vi "Angle Rotation (array).vi"(7 "angle units":T1 items=["radian in, radian out", "radian in, degree out", "degree in, degree out", "degree in, radian out"], 9 "rotated angle range":T2=1 items=["none", "-180 to 180 (-pi to pi)", "0 to 360 (0 to 2pi)"], 10 "Counterclockwise Rotation":dbl[](array[numeric]), 11 "Angle":dbl[](array[numeric])) -> (0 "error":i32, 3 "Rotated Angle":dbl[](array[numeric]))   [LabVIEW 2017, in "NI_AAL_Angle.lvlib"]
doc: "Rotates the input angle counterclockwise.\n\nWire data to the angle input to determine the polymorphic instance to use or manually select the instance."
uses:
  <vilib>/Analysis/NI_AAL_Angle.lvlib
  <vilib>/Analysis/coordinate.llb/Angle Range (Degree).ctl
  <vilib>/Analysis/coordinate.llb/Angle Units.ctl
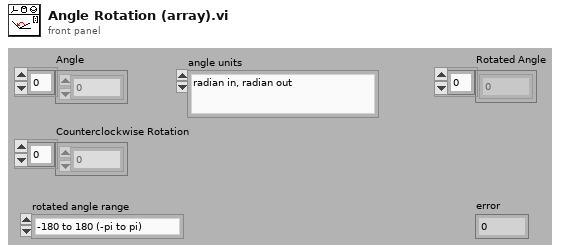
[diagram p1: front panel]
types:
  T1 = typedef "NI_AAL_Angle.lvlib/Angle Units.ctl" = i32
  T2 = typedef "NI_AAL_Angle.lvlib/Angle Range (Degree).ctl" = u16
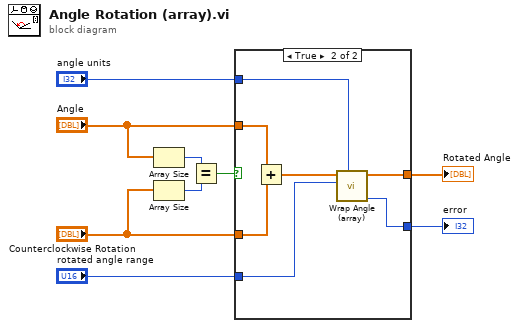
[diagram p0: block diagram]
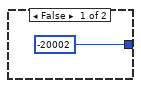
[diagram p2: hidden frame]
diagram:
  n1 = Array Size(array="Angle") -> (size(s)=w9:i32)
  n2 = Array Size(array="Counterclockwise Rotation") -> (size(s)=w8:i32)
  n3 = Equal?(x=w9, y=w8) -> (x = y?=w7:bool)
  n4 = case shown="True" w7 {
    tunnel: "Counterclockwise Rotation" -> [_ w16]
    tunnel: "Angle" -> [_ w17]
    tunnel: "rotated angle range" -> [_ w14]
    tunnel: [_ w13] -> w3
    tunnel: [-20002 ("error") w12] -> w2
    tunnel: "angle units" -> [_ w11]
    frame False {
    }
    frame True {
      n5 = Add(x=w17, y=w16) -> (x+y=w15:dbl[])
      n6 = call <vilib>:"Wrap Angle (array).vi"("angle units"=w11, "angle range"=w14, "Angle In"=w15) -> ("error"=w12:i32, "Angle Out"=w13:dbl[])  [unwired: 7 in]
    }
  }
  "Rotated Angle" <- w3
  "error" <- w2
